vi "Xbox Conversion.vi"(11 "Joystick Values":T2) -> (3 "Driver":T3)   [LabVIEW 2012]
uses:
  <vilib>/Rock Robotics/WPI/Joystick/WPI_JoystickButtonState.ctl
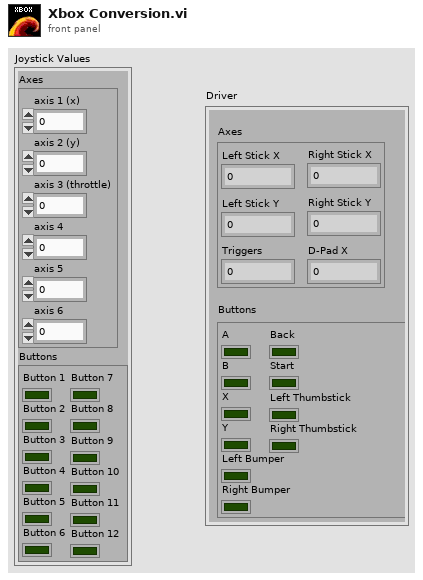
[diagram p1: front panel]
types:
  T1 = typedef "WPI_JoystickButtonState.ctl" = cluster{"Button 1":bool, "Button 2":bool, "Button 3":bool, "Button 4":bool, "Button 5":bool, "Button 6":bool, "Button 7":bool, "Button 8":bool, "Button 9":bool, "Button 10":bool, "Button 11":bool, "Button 12":bool}
  T2 = cluster{"Axes":cluster{"axis 1 (x)":dbl, "axis 2 (y)":dbl, "axis 3 (throttle)":dbl, "axis 4":dbl, "axis 5":dbl, "axis 6":dbl}, "Buttons":T1}
  T3 = cluster{"Buttons":cluster{"A":bool, "B":bool, "X":bool, "Y":bool, "Left Bumper":bool, "Right Bumper":bool, "Back":bool, "Start":bool, "Left Thumbstick":bool, "Right Thumbstick":bool}, "Axes":cluster{"Left Stick X ":dbl, "Left Stick Y":dbl, "Triggers":dbl, "Right Stick X":dbl, "Right Stick Y":dbl, "D-Pad X":dbl}}
  T4 = cluster{"axis 1 (x)":dbl, "axis 2 (y)":dbl, "axis 3 (throttle)":dbl, "axis 4":dbl, "axis 5":dbl, "axis 6":dbl}
  T5 = cluster{"A":bool, "B":bool, "X":bool, "Y":bool, "Left Bumper":bool, "Right Bumper":bool, "Back":bool, "Start":bool, "Left Thumbstick":bool, "Right Thumbstick":bool}
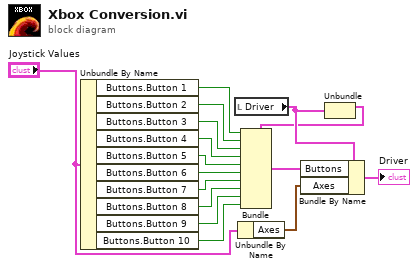
[diagram p0: block diagram]
diagram:
  n1 = Unbundle By Name("Joystick Values") -> ("Buttons.Button 1"=w7:bool, "Buttons.Button 2"=w8:bool, "Buttons.Button 3"=w9:bool, "Buttons.Button 4"=w10:bool, "Buttons.Button 5"=w11:bool, "Buttons.Button 6"=w12:bool, "Buttons.Button 7"=w13:bool, "Buttons.Button 8"=w14:bool, "Buttons.Button 9"=w15:bool, "Buttons.Button 10"=w5:bool)
  n2 = local read "Driver"() -> (w3:T3)
  n3 = Unbundle By Name("Joystick Values") -> ("Axes"=w4:T4)
  n4 = Unbundle(w3) -> ("Buttons"=w2:T5)  [unwired: 1 out]
  n5 = Bundle(cluster=w2, "A"=w7, "B"=w8, "X"=w9, "Y"=w10, "Left Bumper"=w11, "Right Bumper"=w12, "Back"=w13, "Start"=w14, "Left Thumbstick"=w15, "Right Thumbstick"=w5) -> (w6:T5)
  n6 = Bundle By Name(cluster=w3, "Buttons"=w6, "Axes"=w4) -> (→"Driver":T3)
